vi "Initialize Object Map.vi"(8 "error in":errorcluster, 9 "object name":string, 10 "incoming objects":map{string, map{string, i32}}(c390), 11 "object map in":T1) -> (0 "error out":errorcluster, 3 "object map out":T1)   [LabVIEW 2019, in "HLA Custom Device Engine.lvlib"]
uses:
  HLA Custom Device Engine.lvlib
  map_object_value.ctl
  map_attr_param_data.ctl
  emea-ni-adg-hla-lv/src/helpers/Attribute Handle Set/ahs.lvlib
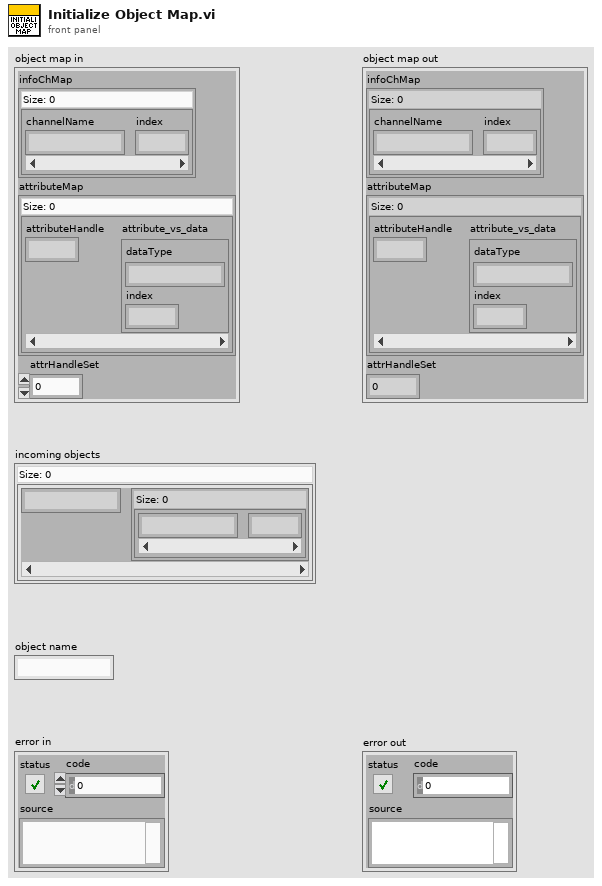
[diagram p1: front panel]
types:
  T1 = typedef "HLA Custom Device Engine.lvlib/map_object_value.ctl" = cluster{"infoChMap":map{string, i32}, "attributeMap":map{u64, T2}, "attrHandleSet":u64}
  T2 = typedef "HLA Custom Device Engine.lvlib/map_attr_param_data.ctl" = cluster{"dataType":string, "index":i32}
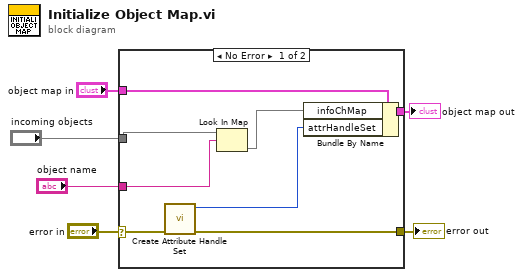
[diagram p0: block diagram]
diagram:
  n1 = case shown="No Error" "error in" {
    selector: "error in" -> [w9 w16]
    tunnel: "object name" -> [w14 _]
    tunnel: [w13 w15] -> w5
    tunnel: "object map in" -> [w11 w15]
    tunnel: "incoming objects" -> [w10 _]
    tunnel: [w8 w16] -> w1
    frame No Error {
      n2 = call "Create Attribute Handle Set.vi"("error in"=w9) -> ("error out"=w8:errorcluster, "attrHandleSet"=w7:u64)  [unwired: 9 in]
      n3 = Look In Map(map=w10, key=w14) -> (value=w12:map{string, i32})  [unwired: 1 in, 1 out]
      n4 = Bundle By Name(cluster=w11, "infoChMap"=w12, "attrHandleSet"=w7) -> (w13:T1)
    }
    frame Error {
    }
  }
  "object map out" <- w5
  "error out" <- w1
